vi "WriteSizeMat_Anything.vi"(6 "Channel":i32=1, 8 "error in":errorcluster, 9 "Height":i32, 10 "Width":i32, 11 "Datatype":refnum<class "Anything.lvclass">) -> (0 "error out":errorcluster, 3 "Datatype":refnum<class "Anything.lvclass">)   [LabVIEW 2020, in "OpenLvVision_OpenCv.lvlib"]
doc: "Write size of the datatype\nNo malleable to breake vi inlining!"
uses:
  OpenLvVision_OpenCv.lvlib
  Anything.lvclass
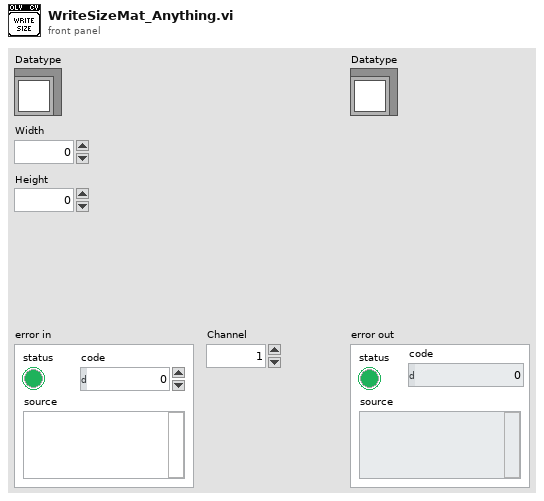
[diagram p1: front panel]
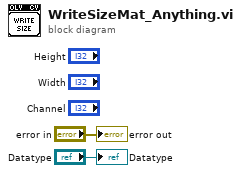
[diagram p0: block diagram]
diagram:
  "error out" <- "error in"
  "Datatype" <- "Datatype"
